vi "cRio Main.vi"() -> ()   [LabVIEW 2009]
uses:
  UDP Lib/UDP Network Location.ctl
panel:
  out "Speed":string
  out "Turn Radius":string
  out "Network Location":T1
  out "End loop":bool
  in  "STOP":bool
  in  "MC VISA resource in":refnum<visa-resource-name>="COM3"
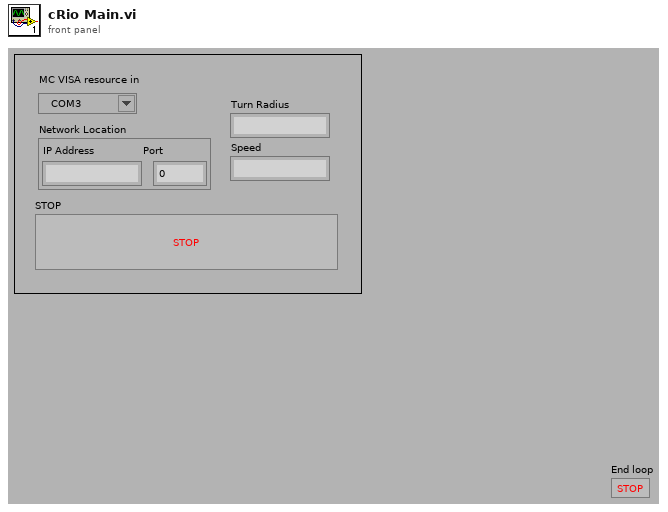
[diagram p1: front panel]
types:
  T1 = typedef "UDP Network Location.ctl" = cluster{"IP Address":string, "Port":u16}
  T2 = typedef "UDP Base.ctl" = cluster{"UDP Session":refnum<k16>, "UDP Socket Params":T3}
  T3 = typedef "UDP Socket Params.ctl" = cluster{"Local Port":u16, "Read Timeout":i32, "Write Timeout":i32}
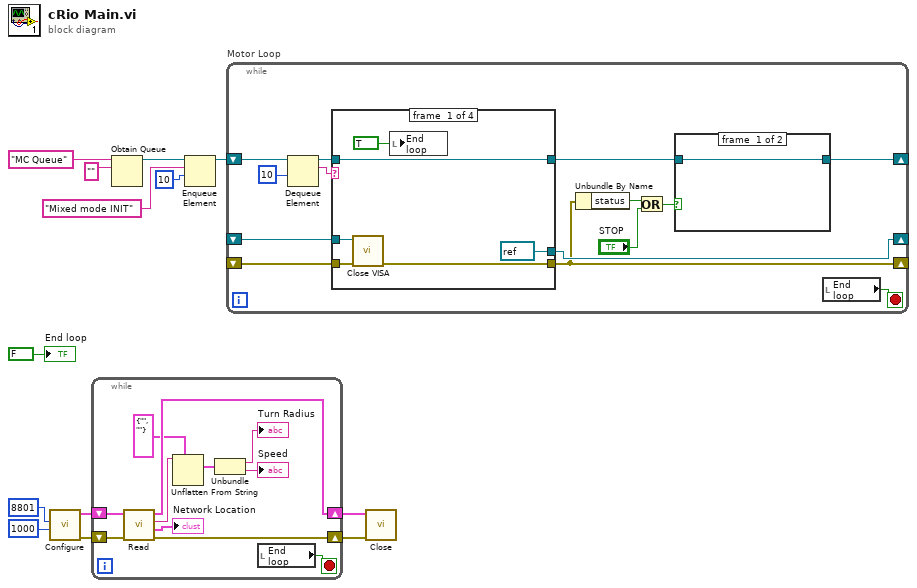
[diagram p0: block diagram]
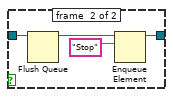
[diagram p2: hidden frame]
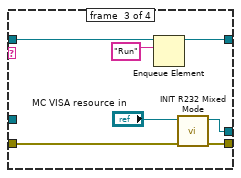
[diagram p4: hidden frame]
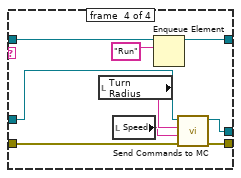
[diagram p5: hidden frame]
diagram:
  n1 = call "Configure.vi"("Read Timeout"=1000, "Local Port"=u16 8801) -> ("error out"=w5:errorcluster, "UDP Base out"=w6:T2)  [unwired: 8 in]
  n2 = while {
    shift-right: [w22] -> w3
    shift-left: w6 -> [w24]
    shift-right: [w14] -> w1
    shift-left: w5 -> [w23]
    stop <- w20 stop-if-true
    n3 = call "Read.vi"("error in (no error)"=w23, "UDP Base in"=w24) -> ("error out"=w14:errorcluster, "Network Location"=→"Network Location":T1, "Receive Data"=w19:string, "UDP Base out"=w22:T2)  [unwired: 4 in, 2 out]
    n4 = Unflatten From String(type=cluster{"element":string, "element":string} {"element"="", "element"=""} ("output cluster"), binary string=w19) -> (value=w17:cluster{"element":string, "element":string})  [unwired: 3 in, 2 out]
    n5 = Unbundle(w17) -> ("element"=→"Turn Radius":string, "element"=→"Speed":string)
    n6 = local read "End loop"() -> (w20:bool)
  }
  n7 = Obtain Queue(name (unnamed)="MC Queue", element data type="" ("name (unnamed)")) -> (queue out=w13:refnum<queue>)  [unwired: 3 in, 2 out]
  n8 = Enqueue Element(queue=w13, element="Mixed mode INIT", timeout in ms (-1)=10) -> (queue out=w9:refnum<queue>)  [unwired: 1 in, 2 out]
  n9 = while "Motor Loop" {
    shift-right: [w26] -> _
    shift-left: w9 -> [w36]
    shift-right: [w34] -> _
    shift-left: _ -> [w33]
    shift-right: [w31] -> _
    shift-left: _ -> [w32]
    stop <- w25 stop-if-true
    n10 = Dequeue Element(queue=w36, timeout in ms (-1)=10) -> (queue out=w35:refnum<queue>, element=w38:string)  [unwired: 1 in, 2 out]
    n11 = case shown="\"Mixed mode INIT\"" w38 {
      tunnel: w35 -> [w46 w52 w58 w67]
      tunnel: [w46 w52 w59 w68] -> w27
      tunnel: [refnum<visa-resource-name> refnum ("MC refrence out") w51 w56 w66] -> w34
      tunnel: [w49 w50 w55 w65] -> w31
      tunnel: w33 -> [w47 w51 _ w64]
      tunnel: w32 -> [w48 w50 w53 w63]
      frame #0 {
        n12 = call "Close VISA.vi"("MC error in"=w48, "MC VISA resource"=w47) -> ("MC error out"=w49:errorcluster)  [unwired: 9 in]
        n13 = local write "End loop"(TRUE ("End loop")) -> ()
      }
      frame #1 {
      }
      frame #2 {
        n14 = Enqueue Element(queue=w58, element="Run") -> (queue out=w59:refnum<queue>)  [unwired: 2 in, 2 out]
        n15 = call "INIT R232 Mixed Mode.vi"("error in (no error)"=w53, "MC VISA resource in"="MC VISA resource in") -> ("MC error out"=w55:errorcluster, "MC VISA resource  out"=w56:refnum<visa-resource-name>)  [unwired: 8 in]
      }
      frame #3 {
        n16 = local read "Turn Radius"() -> (w61:string)
        n17 = local read "Speed"() -> (w60:string)
        n18 = Enqueue Element(queue=w67, element="Run") -> (queue out=w68:refnum<queue>)  [unwired: 2 in, 2 out]
        n19 = call "Send Commands to MC.vi"("error in"=w63, 6:w60, 7:w61, "MC refrence in"=w64) -> ("error out"=w65:errorcluster, "MC refrence out"=w66:refnum<visa-resource-name>)  [unwired: 3 in]
      }
    }
    n20 = Unbundle By Name(w31) -> ("status"=w30:bool)
    n21 = Or(x=w30, y="STOP") -> (x .or. y?=w28:bool)
    n22 = case shown="True" w28 {
      tunnel: w27 -> [w39 w43]
      tunnel: [w39 w41] -> w26
      frame #0 {
      }
      frame #1 {
        n23 = Flush Queue(queue=w43) -> (queue out=w42:refnum<queue>)  [unwired: 1 in, 2 out]
        n24 = Enqueue Element(queue=w42, element="Stop") -> (queue out=w41:refnum<queue>)  [unwired: 2 in, 2 out]
      }
    }
    n25 = local read "End loop"() -> (w25:bool)
  }
  n26 = call "Close.vi"("error in (no error)"=w1, "Cluster of class private data"=w3) -> ()  [unwired: 9 in, 1 out]
  "End loop" <- FALSE ("End loop")
